vi "Execute Query SQLServer.vi"(8 "error in (no error)":errorcluster, 10 "Query":string, 11 "ADODB._Connection":refnum<k7>) -> (0 "error out":errorcluster, 1 "element":string, 2 "Record Affected":i32, 3 "ADODB._Connection 2":refnum<k7>, 4 "No.of Row":i32, 5 "Data":string[][](array[string]))   [LabVIEW 2017]
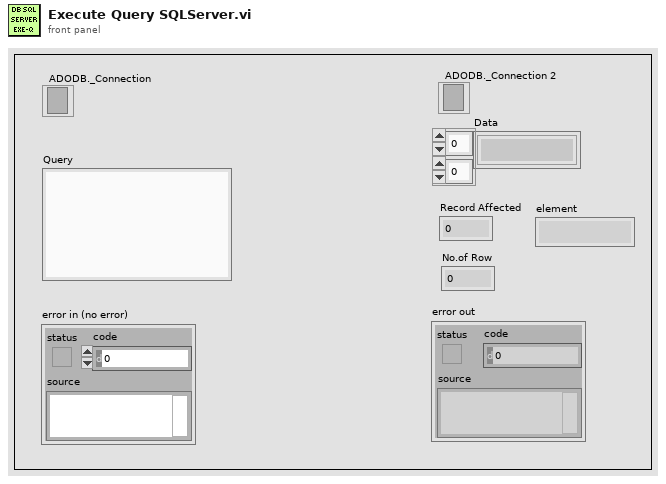
[diagram p1: front panel]
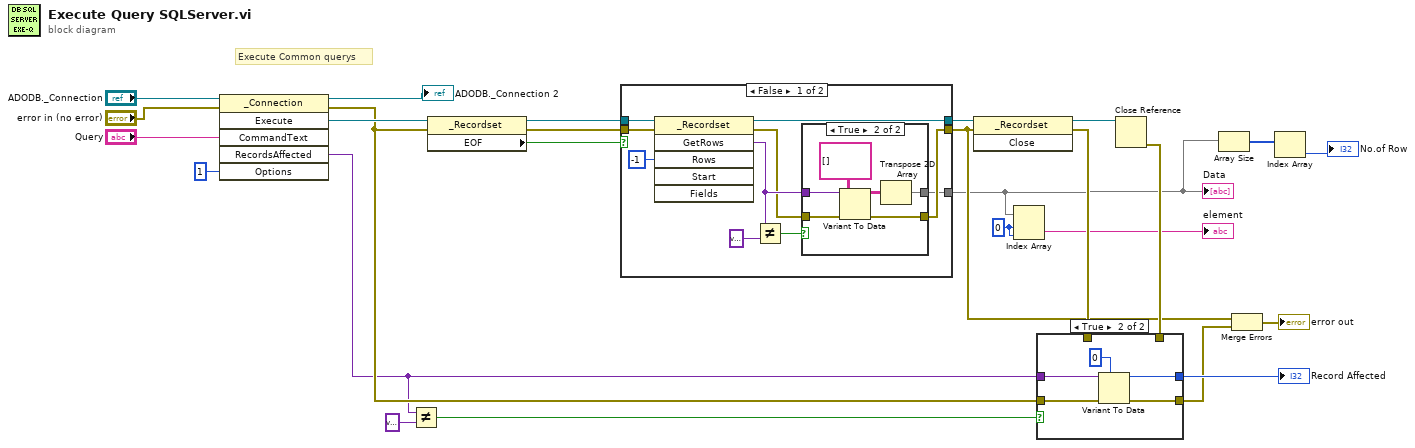
[diagram p0: block diagram]
diagram:
  w9 = 0 ("index (row)")
  # "Execute Common querys"
  n1 = invoke class="_Connection" method="Execute"(reference="ADODB._Connection", error in="error in (no error)", "CommandText"="Query", "Options"=1) -> (reference out=→"ADODB._Connection 2":refnum<k7>, error out=w17:errorcluster, "Execute"=w18:refnum<k7>, "RecordsAffected"=w4:variant)  [unwired: 2 in, 2 out]
  n2 = Not Equal?(x=w4, y=variant) -> (x != y?=w23:bool)
  n3 = property class="_Recordset"(reference=w18, error in=w17) -> (reference out=w15:refnum<k7>, error out=w14:errorcluster, "EOF"=w16:bool)
  n4 = case shown="False" w16 {
    tunnel: w15 -> [w35 w45]
    tunnel: w14 -> [w34 w44]
    tunnel: [w33 w45] -> w13
    tunnel: [w28 w44] -> w12
    tunnel: [w27 _] -> w3
    frame False {
      n5 = invoke class="_Recordset" method="GetRows"(reference=w35, error in=w34, "Rows"=-1) -> (reference out=w33:refnum<k7>, error out=w29:errorcluster, "GetRows"=w30:variant)  [unwired: 3 in, 3 out]
      n6 = Not Equal?(x=w30, y=variant) -> (x != y?=w31:bool)
      n7 = case shown="True" w31 {
        tunnel: w30 -> [_ w43]
        tunnel: [w37 w42] -> w28
        tunnel: [_ w38] -> w27
        tunnel: w29 -> [w37 w40]
        frame False {
        }
        frame True {
          n8 = Variant To Data(error in=w40, type=string[][] [], Variant=w43) -> (data=w39:string[][], error out=w42:errorcluster)
          n9 = Transpose 2D Array(2D array=w39) -> (transposed array=w38:string[][])
        }
      }
    }
    frame True {
    }
  }
  "Data" <- w3
  n10 = invoke class="_Recordset" method="Close"(reference=w13, error in=w12) -> (reference out=w20:refnum<k7>, error out=w21:errorcluster)  [unwired: 1 in, 1 out]
  n11 = Index Array(array=w3, index (row)=w9, index (col)=w9) -> (element=→"element":string)
  n12 = Close Reference(reference=w20) -> (error out=w19:errorcluster)  [unwired: 1 in]
  n13 = case shown="True" w23 {
    tunnel: w4 -> [_ w50]
    tunnel: w17 -> [w46 w51]
    tunnel: [w46 w48] -> w11
    tunnel: [_ w47] -> w22
    tunnel: w21 -> [_ _]
    tunnel: w19 -> [_ _]
    frame False {
    }
    frame True {
      n14 = Variant To Data(error in=w51, type=0, Variant=w50) -> (data=w47:i32, error out=w48:errorcluster)
    }
  }
  "Record Affected" <- w22
  n15 = Array Size(array=w3) -> (size(s)=w2:i32[])
  n16 = Merge Errors(w12, w11) -> (→"error out":errorcluster)
  n17 = Index Array(array=w2) -> (element=→"No.of Row":i32)  [unwired: 1 in]
